vi "FL_Calculate_phi_theta_etc_array.vi"(0 "sin(a)":sgl[](array[numeric]), 1 "R from center":sgl[](array[numeric]), 2 "Mouse Xc":sgl[](array[numeric]), 3 "Mouse Yc":sgl[](array[numeric]), 4 "X1-X2":sgl[](array[numeric]), 5 "Y1-Y2":sgl[](array[numeric])) -> (13 "Mouse-angle":dbl[](array[numeric]), 14 "phi":dbl[](array[numeric]), 15 "Mouse-wall angle":dbl[](array[numeric]), 16 "Rel X":dbl[](array[numeric]), 17 "Rel Y":dbl[](array[numeric]), 18 "From center towards mouse":dbl[](array[numeric]), 19 "Cage rotation angle":sgl[](array[numeric]))   [LabVIEW 2018, in "Tracker.lvlib"]
uses:
  Tracker.lvlib
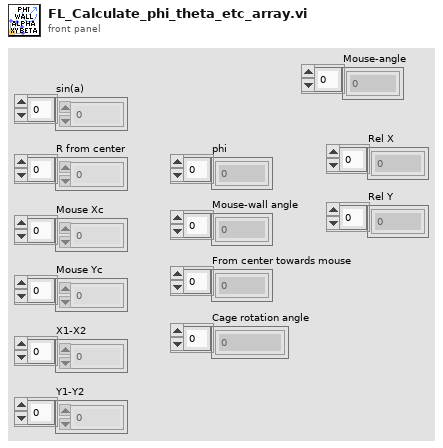
[diagram p1: front panel]
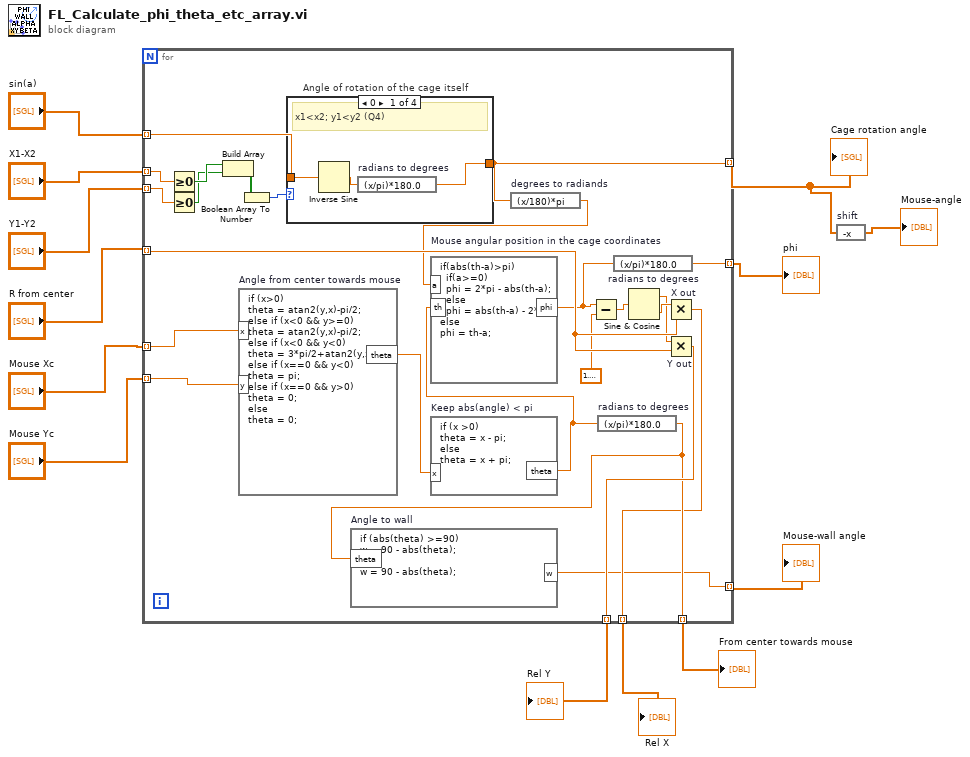
[diagram p0: block diagram]
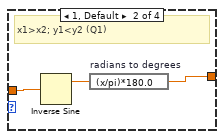
[diagram p2: hidden frame]
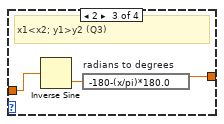
[diagram p3: hidden frame]
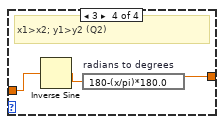
[diagram p4: hidden frame]
diagram:
  n1 = for {
    tunnel: "X1-X2" -> [w37] mode=indexing
    tunnel: "Y1-Y2" -> [w36] mode=indexing
    tunnel: "sin(a)" -> [w31] mode=indexing
    tunnel: [w27] -> w2 mode=indexing
    tunnel: "Mouse Xc" -> [w29] mode=indexing
    tunnel: "Mouse Yc" -> [w30] mode=indexing
    tunnel: "R from center" -> [w26] mode=indexing
    tunnel: [w15] -> w7 mode=indexing
    tunnel: [w28] -> w8 mode=indexing
    tunnel: [w14] -> w3 mode=indexing
    tunnel: [w21] -> w9 mode=indexing
    tunnel: [w25] -> w4 mode=indexing
    n2 = Greater Or Equal To 0?(x=w37) -> (x >= 0?=w35:bool)
    n3 = Greater Or Equal To 0?(x=w36) -> (x >= 0?=w34:bool)
    n4 = Build Array(w35, w34) -> (w33:bool[])
    n5 = formula code="if (x>0)\ntheta = atan2(y,x)-pi/2;\nelse if (x<0 && y>=0)\ntheta = atan2(y,x)-pi/2;\nelse if (x<0 && y<0)\ntheta = 3*pi/2+atan2(y,x);\nelse if (x==0 && y<0)\ntheta = pi;\nelse if (x==0 && y>0)\ntheta = 0;\nelse\ntheta = 0;" "Angle from center towards mouse"("x"=w29, "y"=w30) -> ("theta"=w24:dbl)
    n6 = Boolean Array To Number(Boolean array=w33) -> (number=w32:u32)
    n7 = case "Angle of rotation of the cage itself" shown="0" w32 {
      tunnel: w31 -> [w39 w42 w45 w48]
      tunnel: [w38 w41 w44 w47] -> w27
      frame 0 {
        # "x1<x2; y1<y2 (Q4)"
        n8 = Inverse Sine(1:w39) -> (0:w40:sgl)
        n9 = expression code="(x/pi)*180.0" "radians to degrees"(w40) -> (w38:sgl)
      }
      frame 1, Default {
        # "x1>x2; y1<y2 (Q1)"
        n10 = Inverse Sine(1:w42) -> (0:w43:sgl)
        n11 = expression code="(x/pi)*180.0" "radians to degrees"(w43) -> (w41:sgl)
      }
      frame 2 {
        # "x1<x2; y1>y2 (Q3)"
        n12 = Inverse Sine(1:w45) -> (0:w46:sgl)
        n13 = expression code="-180-(x/pi)*180.0" "radians to degrees"(w46) -> (w44:sgl)
      }
      frame 3 {
        # "x1>x2; y1>y2 (Q2)"
        n14 = Inverse Sine(1:w48) -> (0:w49:sgl)
        n15 = expression code="180-(x/pi)*180.0" "radians to degrees"(w49) -> (w47:sgl)
      }
    }
    n16 = formula code="if (x >0)\ntheta = x - pi;\nelse\ntheta = x + pi;" "Keep abs(angle) < pi"("x"=w24) -> ("theta"=w20:dbl)
    n17 = expression code="(x/180)*pi" "degrees to radiands"(w27) -> (w19:sgl)
    n18 = formula code="if(abs(th-a)>pi)\n  if(a>=0)\n  phi = 2*pi - abs(th-a);\n  else\n  phi = abs(th-a) - 2*pi;\nelse\nphi = th-a;" "Mouse angular position in the cage coordinates"("th"=w20, "a"=w19) -> ("phi"=w17:dbl)
    n19 = Subtract(x=w17, y=1.5707963267948966) -> (x-y=w18:dbl)
    n20 = expression code="(x/pi)*180.0" "radians to degrees"(w20) -> (w21:dbl)
    n21 = formula code="if (abs(theta) >=90)\nw = 90 - abs(theta);\nelse\nw = 90 - abs(theta);" "Angle to wall"("theta"=w21) -> ("w"=w14:dbl)
    n22 = expression code="(x/pi)*180.0" "radians to degrees"(w17) -> (w25:dbl)
    n23 = Sine & Cosine(0:w18) -> (1:w22:dbl, 2:w23:dbl)
    n24 = Multiply "X out"(x=w23, y=w26) -> (x*y=w15:dbl)
    n25 = Multiply "Y out"(x=w22, y=w26) -> (x*y=w28:dbl)
  }
  "Cage rotation angle" <- w2
  "Mouse-wall angle" <- w3
  "From center towards mouse" <- w9
  "phi" <- w4
  "Rel Y" <- w8
  "Rel X" <- w7
  n26 = expression code="-x" "shift"(w2) -> (→"Mouse-angle":sgl[])
